vi "Syntax Check & RPN.vi"(8 "error in (no error)":errorcluster, 11 "STEP in":refnum<class "STEP.lvclass">) -> (0 "error out":errorcluster, 3 "STEP out":refnum<class "STEP.lvclass">)   [LabVIEW 2014, in "SeqLoop.lvlib" / "STEP Classes.lvlib" / "STEP.lvclass"]
uses:
  STEP.lvclass
  STEP.lvclass/STEP.ctl
  SeqLoop.lvlib
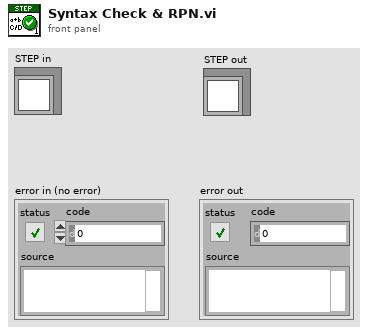
[diagram p1: front panel]
types:
  T1 = typedef "SeqLoop.lvlib/LogicParsedExpression.ctl" = cluster{"RPN ":string[], "Variables":string[], "Ctes":string[], "Formula":string, "Message":string}
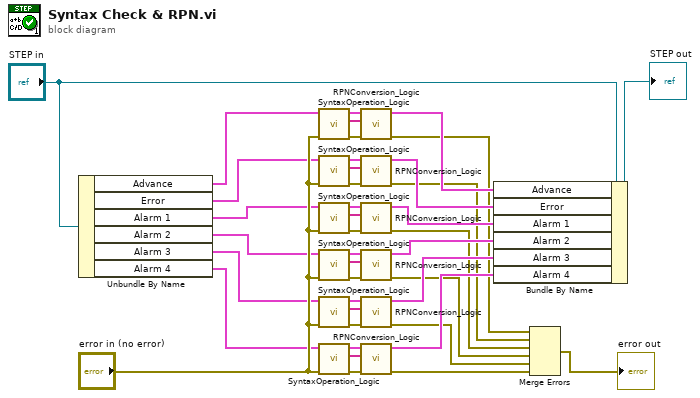
[diagram p0: block diagram]
diagram:
  n1 = Unbundle By Name("STEP in") -> ("Advance"=w2:T1, "Error"=w3:T1, "Alarm 1"=w4:T1, "Alarm 2"=w5:T1, "Alarm 3"=w6:T1, "Alarm 4"=w7:T1)
  n2 = call "SyntaxOperation_Logic.vi"("error in (no error)"="error in (no error)", "Logical Parsed Expression"=w2) -> ("error out"=w9:errorcluster, "Token"=w8:string[], "Logical Parsed Expression Out"=w1:T1)  [unwired: 6 in, 1 out]
  n3 = call "SyntaxOperation_Logic.vi"("error in (no error)"="error in (no error)", "Logical Parsed Expression"=w3) -> ("error out"=w12:errorcluster, "Token"=w11:string[], "Logical Parsed Expression Out"=w10:T1)  [unwired: 6 in, 1 out]
  n4 = call "SyntaxOperation_Logic.vi"("error in (no error)"="error in (no error)", "Logical Parsed Expression"=w4) -> ("error out"=w13:errorcluster, "Token"=w15:string[], "Logical Parsed Expression Out"=w14:T1)  [unwired: 6 in, 1 out]
  n5 = call "SyntaxOperation_Logic.vi"("error in (no error)"="error in (no error)", "Logical Parsed Expression"=w5) -> ("error out"=w18:errorcluster, "Token"=w17:string[], "Logical Parsed Expression Out"=w16:T1)  [unwired: 6 in, 1 out]
  n6 = call "SyntaxOperation_Logic.vi"("error in (no error)"="error in (no error)", "Logical Parsed Expression"=w6) -> ("error out"=w21:errorcluster, "Token"=w20:string[], "Logical Parsed Expression Out"=w19:T1)  [unwired: 6 in, 1 out]
  n7 = call "SyntaxOperation_Logic.vi"("error in (no error)"="error in (no error)", "Logical Parsed Expression"=w7) -> ("error out"=w24:errorcluster, "Token"=w23:string[], "Logical Parsed Expression Out"=w22:T1)  [unwired: 6 in, 1 out]
  n8 = call "RPNConversion_Logic.vi"("error in"=w9, "Token"=w8, "Logical Parsed Expression"=w1) -> ("error out"=w31:errorcluster, "Logical Parsed Expression Out"=w35:T1)  [unwired: 7 in]
  n9 = call "RPNConversion_Logic.vi"("error in"=w12, "Token"=w11, "Logical Parsed Expression"=w10) -> ("error out"=w30:errorcluster, "Logical Parsed Expression Out"=w36:T1)  [unwired: 7 in]
  n10 = call "RPNConversion_Logic.vi"("error in"=w13, "Token"=w15, "Logical Parsed Expression"=w14) -> ("error out"=w29:errorcluster, "Logical Parsed Expression Out"=w37:T1)  [unwired: 7 in]
  n11 = call "RPNConversion_Logic.vi"("error in"=w18, "Token"=w17, "Logical Parsed Expression"=w16) -> ("error out"=w28:errorcluster, "Logical Parsed Expression Out"=w38:T1)  [unwired: 7 in]
  n12 = call "RPNConversion_Logic.vi"("error in"=w21, "Token"=w20, "Logical Parsed Expression"=w19) -> ("error out"=w27:errorcluster, "Logical Parsed Expression Out"=w39:T1)  [unwired: 7 in]
  n13 = call "RPNConversion_Logic.vi"("error in"=w24, "Token"=w23, "Logical Parsed Expression"=w22) -> ("error out"=w26:errorcluster, "Logical Parsed Expression Out"=w40:T1)  [unwired: 7 in]
  n14 = Bundle By Name(cluster="STEP in", "Advance"=w35, "Error"=w36, "Alarm 1"=w37, "Alarm 2"=w38, "Alarm 3"=w39, "Alarm 4"=w40) -> (→"STEP out":refnum<class "STEP.lvclass">)
  n15 = Merge Errors(w31, w30, w29, w28, w27, w26) -> (→"error out":errorcluster)
